vi "PathPlanner_Trajectory25_GenerateStates_Pass1.vi"(8 "StartingRotation":T5={"VALUE"=0.0, "COS"=1.0, "SIN"=0.0} {"SIN" format="%13.4f"; "COS" format="%13.4f"; "VALUE" format="%13.4f"}, 9 "RobotConfig":T1 {"moduleLocations"."Y" format="%14.3f"; "moduleLocations"."X" format="%14.3f"; "ModuleConfig"."driveMotor"."Jr_KgM2" format="%13.5p"; "ModuleConfig"."driveMotor"."L_H" format="%13.5p"; "ModuleConfig"."driveMotor"."Kt_NMPerAmp" format="%13.5p"; "ModuleConfig"."driveMotor"."KvINV_RadPerSecPerVolt" format="%13.5p"; "ModuleConfig"."driveMotor"."R_Ohms" format="%13.5p"; "ModuleConfig"."driveMotor"."FreeSpeed_RadPerSec" format="%13.5p"; "ModuleConfig"."driveMotor"."FreeCurrent_Amps" format="%13.5p"; "ModuleConfig"."driveMotor"."StallCurrent_Amps" format="%13.5p"; "ModuleConfig"."driveMotor"."StallTorque_NM" format="%13.5p"; "ModuleConfig"."driveMotor"."nominalVoltage_Volts" format="%13.5p"}, 10 "in PathPlannerStates":T6[](array[typedef]) {"ModuleStates"."SWERVE_DRIVE_MODULE_STATE"."Angle"."SIN" format="%13.4f"; "ModuleStates"."SWERVE_DRIVE_MODULE_STATE"."Angle"."COS" format="%13.4f"; "ModuleStates"."SWERVE_DRIVE_MODULE_STATE"."Angle"."VALUE" format="%13.4f"; "ModuleStates"."FieldAngle"."SIN" format="%13.4f"; "ModuleStates"."FieldAngle"."COS" format="%13.4f"; "ModuleStates"."FieldAngle"."VALUE" format="%13.4f"; "ModuleStates"."FieldPos"."Y" format="%14.3f"; "ModuleStates"."FieldPos"."X" format="%14.3f"; "DeltaRot"."SIN" format="%13.4f"; "DeltaRot"."COS" format="%13.4f"; "DeltaRot"."VALUE" format="%13.4f"; "pose"."ROTATION"."SIN" format="%13.4f"; "pose"."ROTATION"."COS" format="%13.4f"; "pose"."ROTATION"."VALUE" format="%13.4f"; "pose"."TRANSLATION"."Y" format="%14.3f"; "pose"."TRANSLATION"."X" format="%14.3f"; "FieldSpeeds"."vOmega" format="%10.3f"; "FieldSpeeds"."vY" format="%10.3f"; "FieldSpeeds"."vX" format="%10.3f"; "Heading"."SIN" format="%13.4f"; "Heading"."COS" format="%13.4f"; "Heading"."VALUE" format="%13.4f"}, 11 "PathPlannerPath":T13={"Reversed"=FALSE, "RotationTargets"=[], "ConstraintZones"=[], "EventMarkers"=[], "GlobalConstraints"={"MaxVelocityMps;"=0.0, "MaxAccelerationMpsSq;"=0.0, "MaxAngularVelRadPsEc;"=0.0, "MaxAngularAccRadPSecSq"=0.0, "Exists"=FALSE, "Unlimited"=FALSE, "NominalVoltageVolts"=12.0}, "GoalEndState"={"VelocityMPS"=0.0, "Rotation"={"VALUE"=0.0, "COS"=1.0, "SIN"=0.0}}, "AllPoints"=[], "Name"="", "Waypoints"=[], "PointTowardsZones"=[], "IdealStartingState"={"VelocityMPS"=0.0, "Rotation"={"VALUE"=1.0, "COS"=0.0, "SIN"=0.0}}, "IsChoreoPath"=FALSE, "PreventFlipping"=FALSE} {"IdealStartingState"."Rotation"."SIN" format="%13.4f"; "IdealStartingState"."Rotation"."COS" format="%13.4f"; "IdealStartingState"."Rotation"."VALUE" format="%13.4f"; "PointTowardsZones"."TargetPosition"."Y" format="%14.3f"; "PointTowardsZones"."TargetPosition"."X" format="%14.3f"; "PointTowardsZones"."RotationOffset"."SIN" format="%13.4f"; "PointTowardsZones"."RotationOffset"."COS" format="%13.4f"; "PointTowardsZones"."RotationOffset"."VALUE" format="%13.4f"; "Waypoints"."nextControl"."Y" format="%14.3f"; "Waypoints"."nextControl"."X" format="%14.3f"; "Waypoints"."anchor"."Y" format="%14.3f"; "Waypoints"."anchor"."X" format="%14.3f"; "Waypoints"."prevControl"."Y" format="%14.3f"; "Waypoints"."prevControl"."X" format="%14.3f"; "AllPoints"."RotationTarget"."rotation"."SIN" format="%13.4f"; "AllPoints"."RotationTarget"."rotation"."COS" format="%13.4f"; "AllPoints"."RotationTarget"."rotation"."VALUE" format="%13.4f"; "AllPoints"."Position"."Y" format="%14.3f"; "AllPoints"."Position"."X" format="%14.3f"; "GoalEndState"."Rotation"."SIN" format="%13.4f"; "GoalEndState"."Rotation"."COS" format="%13.4f"; "GoalEndState"."Rotation"."VALUE" format="%13.4f"; "RotationTargets"."rotation"."SIN" format="%13.4f"; "RotationTargets"."rotation"."COS" format="%13.4f"; "RotationTargets"."rotation"."VALUE" format="%13.4f"}) -> (3 "out PathPlannerStates":T6[](array[typedef]) {"ModuleStates"."SWERVE_DRIVE_MODULE_STATE"."Angle"."SIN" format="%13.4f"; "ModuleStates"."SWERVE_DRIVE_MODULE_STATE"."Angle"."COS" format="%13.4f"; "ModuleStates"."SWERVE_DRIVE_MODULE_STATE"."Angle"."VALUE" format="%13.4f"; "ModuleStates"."FieldAngle"."SIN" format="%13.4f"; "ModuleStates"."FieldAngle"."COS" format="%13.4f"; "ModuleStates"."FieldAngle"."VALUE" format="%13.4f"; "ModuleStates"."FieldPos"."Y" format="%14.3f"; "ModuleStates"."FieldPos"."X" format="%14.3f"; "DeltaRot"."SIN" format="%13.4f"; "DeltaRot"."COS" format="%13.4f"; "DeltaRot"."VALUE" format="%13.4f"; "pose"."ROTATION"."SIN" format="%13.4f"; "pose"."ROTATION"."COS" format="%13.4f"; "pose"."ROTATION"."VALUE" format="%13.4f"; "pose"."TRANSLATION"."Y" format="%14.3f"; "pose"."TRANSLATION"."X" format="%14.3f"; "FieldSpeeds"."vOmega" format="%10.3f"; "FieldSpeeds"."vY" format="%10.3f"; "FieldSpeeds"."vX" format="%10.3f"; "Heading"."SIN" format="%13.4f"; "Heading"."COS" format="%13.4f"; "Heading"."VALUE" format="%13.4f"})   [LabVIEW 2019, in "PathPlanner24.lvlib"]
doc: "Internal routine to help create a trajectory from a path."
uses:
  PathPlanner24.lvlib
  TypeDef/PathPlannerTrajectoryState25.ctl
  <vilib>/Rock Robotics/WPI/ThirdParty/JAS_Junk/TrajLib/TypeDef/ROTATION2D.ctl
  TypeDef/PathPlannerPathConstraints.ctl
  <vilib>/Rock Robotics/WPI/ThirdParty/JAS_Junk/TrajLib/TypeDef/CHASSIS_SPEEDS.ctl
  <vilib>/Rock Robotics/WPI/ThirdParty/JAS_Junk/TrajLib/TypeDef/POSE2D.ctl
  <vilib>/Rock Robotics/WPI/ThirdParty/JAS_Junk/TrajLib/TypeDef/TRANSLATION2D.ctl
  TypeDef/PathPlannerSwerveModTrajState.ctl
  <vilib>/Rock Robotics/WPI/ThirdParty/JAS_Junk/TrajLib/TypeDef/SWERVE_DRIVE_MODULE_STATE.ctl
  TypeDef/PathPlannerDriveFeedFwds.ctl
  TypeDef/PathPlannerPath.ctl
  TypeDef/PathPlannerRotationTarget.ctl
  TypeDef/PathPlannerConstraintsZone.ctl
  TypeDef/PathPlannerEventMarker.ctl
  TypeDef/PathPlannerCommandUtil.ctl
  ENum/PathPlanner_CommandUtilType_ENUM.ctl
  TypeDef/PathPlannerGoalEndState.ctl
  TypeDef/PathPlannerPathPoint.ctl
  TypeDef/PathPlannerWaypoint.ctl
  TypeDef/PathPlannerPointTowardsZone.ctl
  TypeDef/PathPlannerIdealStartingState.ctl
  TypeDef/PathPlannerRobotConfig.ctl
  TypeDef/PathPlannerModuleConfig.ctl
  <vilib>/Rock Robotics/WPI/ThirdParty/JAS_Junk/TrajLib/TypeDef/DCMOTOR.CTL
  PathPlanner_GeomUtil_RotationLerp.vi
  <vilib>/Rock Robotics/WPI/ThirdParty/JAS_Junk/TrajLib/Translation2d_Create.vi
  <vilib>/Rock Robotics/WPI/ThirdParty/JAS_Junk/TrajLib/Util_CalcDist.vi
  <vilib>/Rock Robotics/WPI/ThirdParty/JAS_Junk/TrajLib/Translation2d_GetXY.vi
  <vilib>/Rock Robotics/WPI/ThirdParty/JAS_Junk/TrajLib/Rotation2d_CreateXY.vi
  <vilib>/Rock Robotics/WPI/ThirdParty/JAS_Junk/TrajLib/Conv_Deg_Radians.vi
  <vilib>/Rock Robotics/WPI/ThirdParty/JAS_Junk/TrajLib/Rotation2d_RotateBy.vi
  <vilib>/Rock Robotics/WPI/ThirdParty/JAS_Junk/TrajLib/Rotation2d_UnaryMinus.vi
  <vilib>/Rock Robotics/WPI/ThirdParty/JAS_Junk/TrajLib/Rotation2d_Times.vi
  <vilib>/Rock Robotics/WPI/ThirdParty/JAS_Junk/TrajLib/Trajectory_Library.lvlib
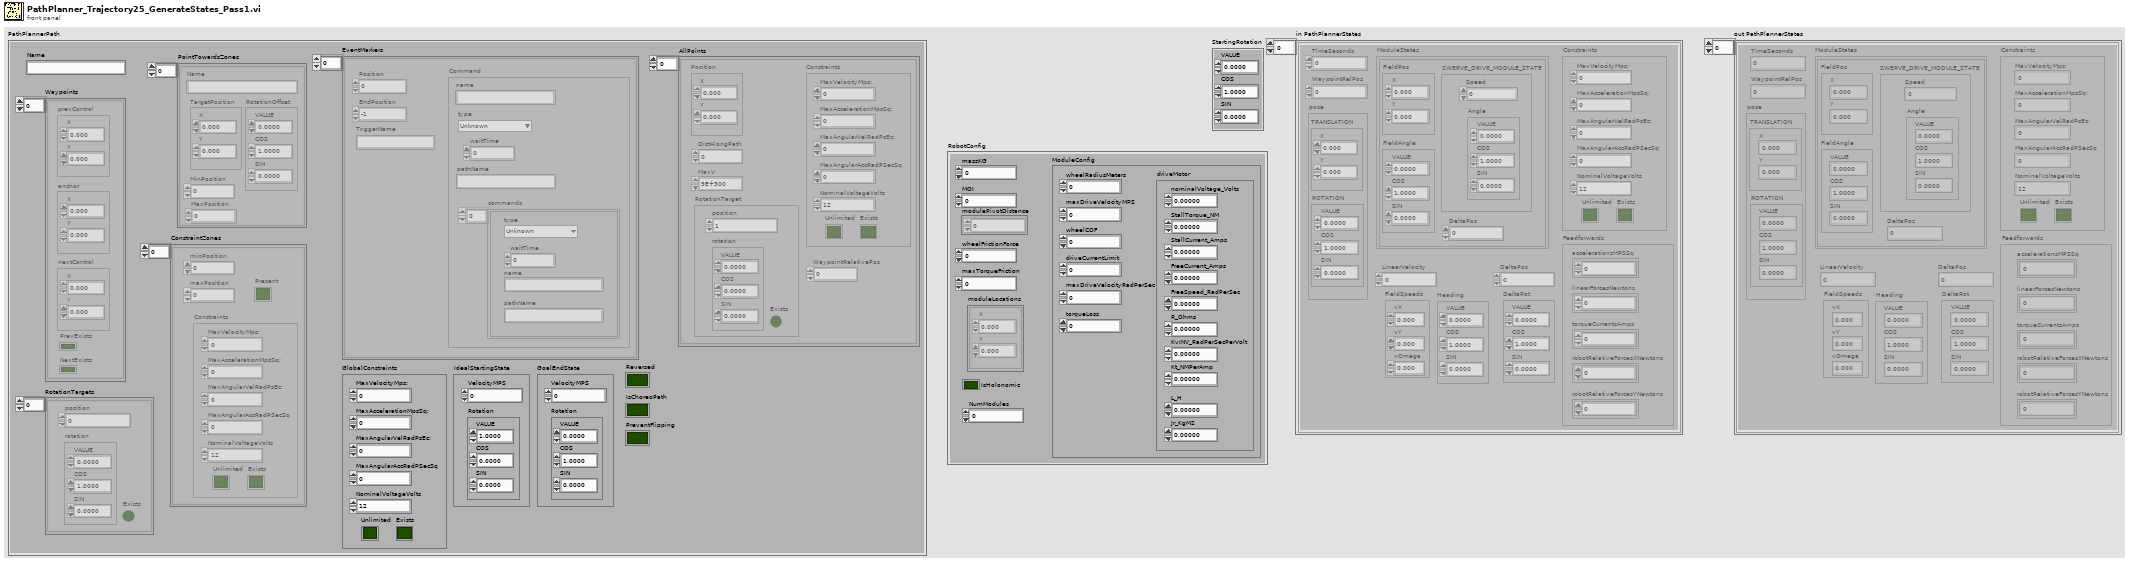
[diagram p1: front panel]
types:
  T1 = typedef "PathPlanner24.lvlib/PathPlannerRobotConfig.ctl" = cluster{"massKG":dbl, "MOI":dbl, "modulePivotDistance":dbl[], "wheelFrictionForce":dbl, "maxTorqueFriction":dbl, "ModuleConfig":T2, "moduleLocations":T4[], "IsHolonomic":bool, "NumModules":i32}
  T2 = typedef "PathPlanner24.lvlib/PathPlannerModuleConfig.ctl" = cluster{"wheelRadiusMeters":dbl, "maxDriveVelocityMPS":dbl, "wheelCOF":dbl, "driveCurrentLimit":dbl, "maxDriveVelocityRadPerSec":dbl, "torqueLoss":dbl, "driveMotor":T3}
  T3 = typedef "Trajectory_Library.lvlib/DCMOTOR.CTL" = cluster{"nominalVoltage_Volts":dbl, "StallTorque_NM":dbl, "StallCurrent_Amps":dbl, "FreeCurrent_Amps":dbl, "FreeSpeed_RadPerSec":dbl, "R_Ohms":dbl, "KvINV_RadPerSecPerVolt":dbl, "Kt_NMPerAmp":dbl, "L_H":dbl, "Jr_KgM2":dbl}
  T4 = typedef "Trajectory_Library.lvlib/TRANSLATION2D.ctl" = cluster{"X":dbl, "Y":dbl}
  T5 = typedef "Trajectory_Library.lvlib/ROTATION2D.ctl" = cluster{"VALUE":dbl, "COS":dbl, "SIN":dbl}
  T6 = typedef "PathPlanner24.lvlib/PathPlannerTrajectoryState25.ctl" = cluster{"TimeSeconds":dbl, "LinearVelocity":dbl, "Heading":T5, "Constraints":T7, "DeltaPos":dbl, "FieldSpeeds":T8, "pose":T9, "DeltaRot":T5, "ModuleStates":T10[], "WaypointRelPos":dbl, "Feedforwards":T12}
  T7 = typedef "PathPlanner24.lvlib/PathPlannerPathConstraints.ctl" = cluster{"MaxVelocityMps;":dbl, "MaxAccelerationMpsSq;":dbl, "MaxAngularVelRadPsEc;":dbl, "MaxAngularAccRadPSecSq":dbl, "Exists":bool, "Unlimited":bool, "NominalVoltageVolts":dbl}
  T8 = typedef "Trajectory_Library.lvlib/CHASSIS_SPEEDS.ctl" = cluster{"vX":dbl, "vY":dbl, "vOmega":dbl}
  T9 = typedef "Trajectory_Library.lvlib/POSE2D.ctl" = cluster{"TRANSLATION":T4, "ROTATION":T5}
  T10 = typedef "PathPlanner24.lvlib/PathPlannerSwerveModTrajState.ctl" = cluster{"FieldPos":T4, "FieldAngle":T5, "DeltaPos":dbl, "SWERVE_DRIVE_MODULE_STATE":T11}
  T11 = typedef "Trajectory_Library.lvlib/SWERVE_DRIVE_MODULE_STATE.ctl" = cluster{"Speed":dbl, "Angle":T5}
  T12 = typedef "PathPlanner24.lvlib/PathPlannerDriveFeedFwds.ctl" = cluster{"accelerationsMPSSq":dbl[], "linearForcesNewtons":dbl[], "torqueCurrentsAmps":dbl[], "robotRelativeForcesXNewtons":dbl[], "robotRelativeForcesYNewtons":dbl[]}
  T13 = typedef "PathPlanner24.lvlib/PathPlannerPath.ctl" = cluster{"Reversed":bool, "RotationTargets":T14[], "ConstraintZones":T15[], "EventMarkers":T16[], "GlobalConstraints":T7, "GoalEndState":T19, "AllPoints":T20[], "Name":string, "Waypoints":T21[], "PointTowardsZones":T22[], "IdealStartingState":T23, "IsChoreoPath":bool, "PreventFlipping":bool}
  T14 = typedef "PathPlanner24.lvlib/PathPlannerRotationTarget.ctl" = cluster{"position":dbl, "rotation":T5, "Exists":bool}
  T15 = typedef "PathPlanner24.lvlib/PathPlannerConstraintsZone.ctl" = cluster{"minPosition":dbl, "maxPosition":dbl, "Constraints":T7, "Present":bool}
  T16 = typedef "PathPlanner24.lvlib/PathPlannerEventMarker.ctl" = cluster{"Position":dbl, "Command":T17, "TriggerName":string, "EndPosition":dbl}
  T17 = typedef "PathPlanner24.lvlib/PathPlannerCommandUtil.ctl" = cluster{"waitTime":dbl, "name":string, "pathName":string, "commands":cluster{"type":T18, "waitTime":dbl, "name":string, "pathName":string}[], "type":T18}
  T18 = typedef "PathPlanner24.lvlib/PathPlanner_CommandUtilType_ENUM.ctl" = enum16{"Unknown", "Wait", "Named", "Path", "Sequential", "Parallel", "Race", "Deadline"}
  T19 = typedef "PathPlanner24.lvlib/PathPlannerGoalEndState.ctl" = cluster{"VelocityMPS":dbl, "Rotation":T5}
  T20 = typedef "PathPlanner24.lvlib/PathPlannerPathPoint.ctl" = cluster{"Position":T4, "DistAlongPath":dbl, "MaxV":dbl, "Constraints":T7, "RotationTarget":T14, "WaypointRelativePos":dbl}
  T21 = typedef "PathPlanner24.lvlib/PathPlannerWaypoint.ctl" = cluster{"prevControl":T4, "anchor":T4, "nextControl":T4, "PrevExists":bool, "NextExists":bool}
  T22 = typedef "PathPlanner24.lvlib/PathPlannerPointTowardsZone.ctl" = cluster{"RotationOffset":T5, "Name":string, "TargetPosition":T4, "MinPosition":dbl, "MaxPosition":dbl}
  T23 = typedef "PathPlanner24.lvlib/PathPlannerIdealStartingState.ctl" = cluster{"VelocityMPS":dbl, "Rotation":T5}
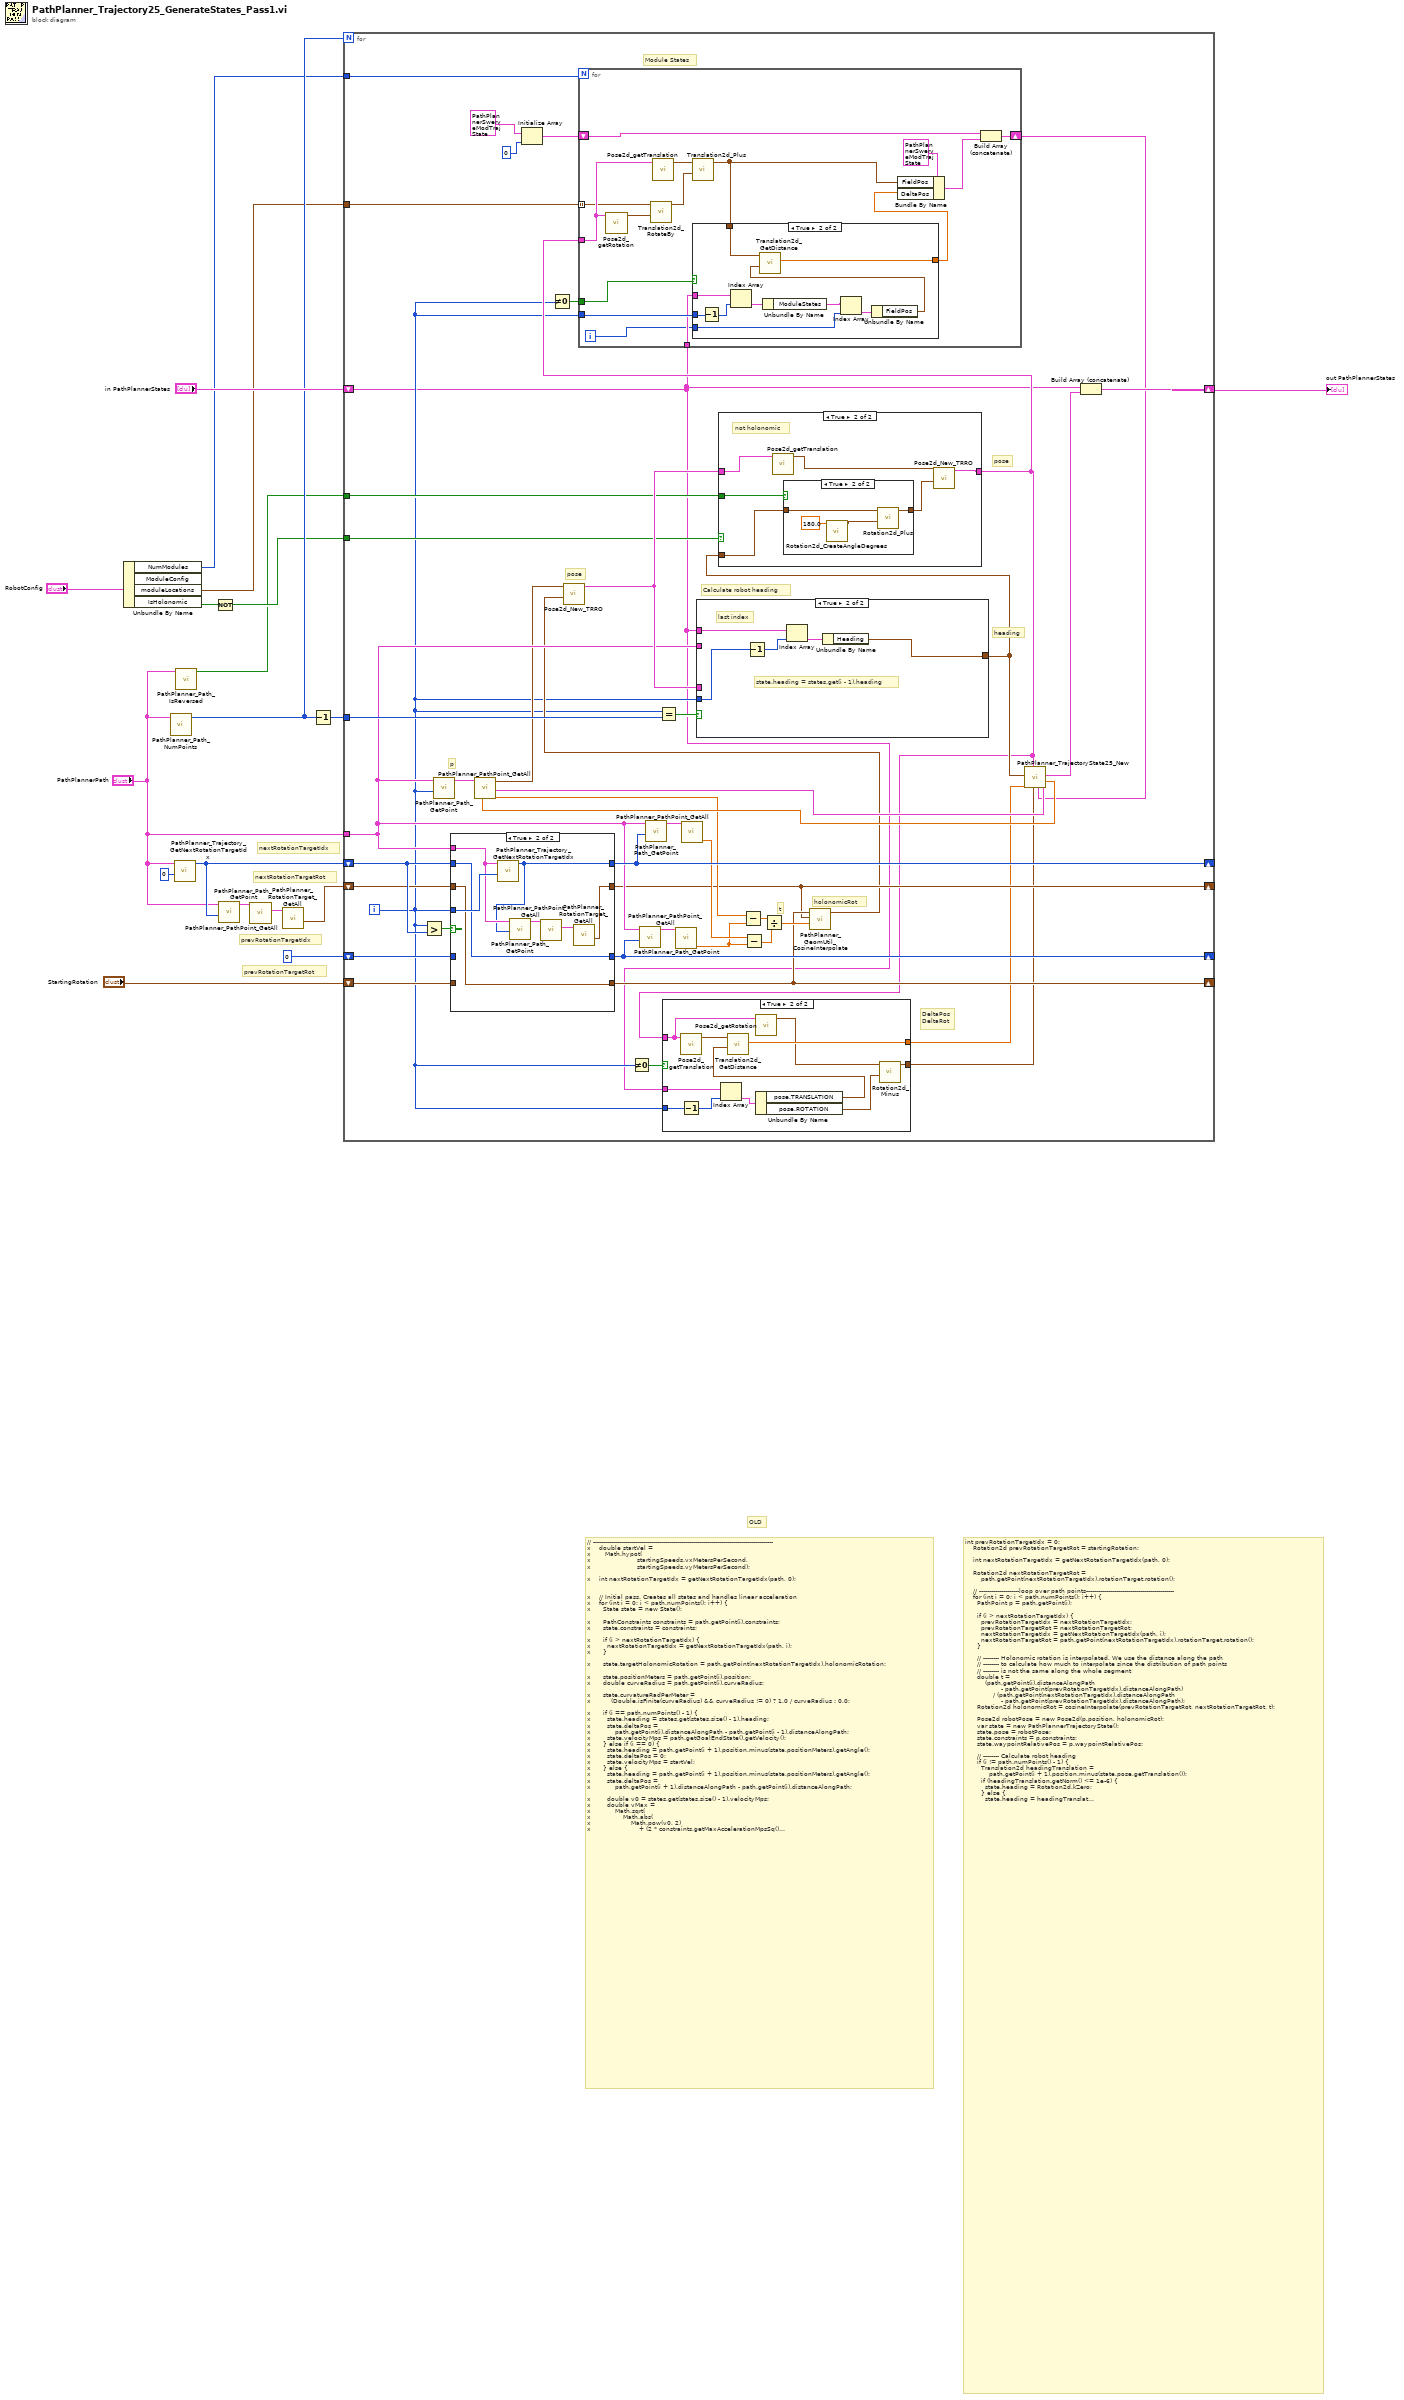
[diagram p0: block diagram]
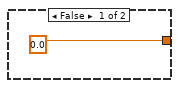
[diagram p2: hidden frame]
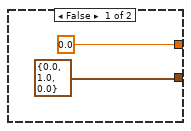
[diagram p3: hidden frame]
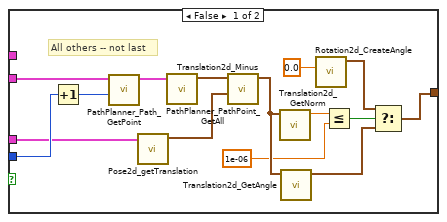
[diagram p6: hidden frame]
diagram:
  # "nextRotationTargetRot"
  # "prevRotationTargetRot"
  # "prevRotationTargetIdx"
  # "nextRotationTargetIdx"
  # "OLD"
  # "int prevRotationTargetIdx = 0;\n    Rotation2d prevRotationTargetRot = startingRotation;\n\n    int nextRotationTargetIdx = getNextRotationTargetIdx(path, 0);\n\n    Rotation2d nextRotationTargetRot =\n        path.getPoint(nextRotationTargetIdx).rotationTarget.rotation();\n\n    // --------------------loop over path points--------------------------------------------\n    for (int i = 0; i < path.numPoints(); i++) {\n      PathPoint p = path.getPoint(i);\n\n      if (i > nextRotationTargetIdx) {\n        prevRotationTargetIdx = nextRotationTargetIdx;\n        prevRotationTargetRot = nextRotationTargetRot;\n        nextRotationTargetIdx = getNextRotationTargetIdx(path, i);\n        nextRotationTargetRot = path.getPoint(nextRotationTargetIdx).rotationTarget.rotation();\n      }\n\n      // -------- Holonomic rotation is interpolated. We use the distance along the path\n      // -------- to calculate how much to interpolate since the distribution of path points\n      // -------- is not the same along the whole segment\n      double t =\n          (path.getPoint(i).distanceAlongPath\n                  - path.getPoint(prevRotationTargetIdx).distanceAlongPath)\n              / (path.getPoint(nextRotationTargetIdx).distanceAlongPath\n                  - path.getPoint(prevRotationTargetIdx).distanceAlongPath);\n      Rotation2d holonomicRot = cosineInterpolate(prevRotationTargetRot, nextRotationTargetRot, t);\n\n      Pose2d robotPose = new Pose2d(p.position, holonomicRot);\n      var state = new PathPlannerTrajectoryState();\n      state.pose = robotPose;\n      state.constraints = p.constraints;\n      state.waypointRelativePos = p.waypointRelativePos;\n\n      // -------- Calculate robot heading\n      if (i != path.numPoints() - 1) {\n        Translation2d headingTranslation =\n            path.getPoint(i + 1).position.minus(state.pose.getTranslation());\n        if (headingTranslation.getNorm() <= 1e-6) {\n          state.heading = Rotation2d.kZero;\n        } else {\n          state.heading = headingTranslation.getAngle();\n        }\n      } else {\n        state.heading = states.get(i - 1).heading;\n      }\n\n      if (!config.isHolonomic) {\n        state.pose =\n            new Pose2d(\n                state.pose.getTranslation(),\n                path.isReversed() ? (state.heading.plus(Rotation2d.k180deg)) : state.heading);\n      }\n\n      if (i != 0) {\n        state.deltaPos =\n            state.pose.getTranslation().getDistance(states.get(i - 1).pose.getTranslation());\n        state.deltaRot = state.pose.getRotation().minus(states.get(i - 1).pose.getRotation());\n      }\n\n      state.moduleStates = new SwerveModuleTrajectoryState[config.numModules];\n      // -------------------------inner loop---------------------------------------\n      for (int m = 0; m < config.numModules; m++) {\n        state.moduleStates[m] = new SwerveModuleTrajectoryState();\n        state.moduleStates[m].fieldPos =\n            state\n                .pose\n                .getTranslation()\n                .plus(config.moduleLocations[m].rotateBy(state.pose.getRotation()));\n\n        if (i != 0) {\n          state.moduleStates[m].deltaPos =\n              state.moduleStates[m].fieldPos.getDistance(\n                  states.get(i - 1).moduleStates[m].fieldPos);\n        }\n      }\n      // ----------------------------end inner loop---------------------------------\n      states.add(state);\n    }\n    // -------------------------------end loop-----------------------------------------------------"
  # "// ------------------------------------------------------------------------------------------\nx    double startVel =\nx       Math.hypot(  \nx                       startingSpeeds.vxMetersPerSecond, \nx                       startingSpeeds.vyMetersPerSecond);\n\nx    int nextRotationTargetIdx = getNextRotationTargetIdx(path, 0);\n\n\nx    // Initial pass. Creates all states and handles linear acceleration\nx    for (int i = 0; i < path.numPoints(); i++) {\nx      State state = new State();\n\nx      PathConstraints constraints = path.getPoint(i).constraints;\nx      state.constraints = constraints;\n\nx      if (i > nextRotationTargetIdx) {\nx        nextRotationTargetIdx = getNextRotationTargetIdx(path, i);\nx      }\n\nx      state.targetHolonomicRotation = path.getPoint(nextRotationTargetIdx).holonomicRotation;\n\nx      state.positionMeters = path.getPoint(i).position;\nx      double curveRadius = path.getPoint(i).curveRadius;\n\nx      state.curvatureRadPerMeter =\nx          (Double.isFinite(curveRadius) && curveRadius != 0) ? 1.0 / curveRadius : 0.0;\n\nx      if (i == path.numPoints() - 1) {\nx        state.heading = states.get(states.size() - 1).heading;\nx        state.deltaPos =\nx            path.getPoint(i).distanceAlongPath - path.getPoint(i - 1).distanceAlongPath;\nx        state.velocityMps = path.getGoalEndState().getVelocity();\nx      } else if (i == 0) {\nx        state.heading = path.getPoint(i + 1).position.minus(state.positionMeters).getAngle();\nx        state.deltaPos = 0;\nx        state.velocityMps = startVel;\nx      } else {\nx        state.heading = path.getPoint(i + 1).position.minus(state.positionMeters).getAngle();\nx        state.deltaPos =\nx            path.getPoint(i + 1).distanceAlongPath - path.getPoint(i).distanceAlongPath;\n\nx        double v0 = states.get(states.size() - 1).velocityMps;\nx        double vMax =\nx            Math.sqrt(\nx                Math.abs(\nx                    Math.pow(v0, 2)\nx                        + (2 * constraints.getMaxAccelerationMpsSq() * state.deltaPos)));\nx        state.velocityMps = Math.min(vMax, path.getPoint(i).maxV);\n      }\n\nX      states.add(state);\n    }"
  n1 = Unbundle By Name("RobotConfig") -> ("NumModules"=w2:i32, "moduleLocations"=w1:T4[], "IsHolonomic"=w6:bool)  [unwired: 1 out]
  n2 = call "PathPlanner_Path_NumPoints.vi"("PathPlannerPath"="PathPlannerPath") -> ("NumPoints"=w14:i32)  [unwired: 10 in]
  n3 = call "PathPlanner_Trajectory_GetNextRotationTargetIdx.vi"("Starting Index"=0, "PathPlannerPath"="PathPlannerPath") -> ("Idx"=w8:i32)  [unwired: 8 in, 1 out]
  n4 = call "PathPlanner_Path_IsReversed.vi"("PathPlannerPath"="PathPlannerPath") -> ("Reversed"=w3:bool)  [unwired: 10 in]
  n5 = Not(x=w6) -> (.not. x?=w5:bool)
  n6 = call "PathPlanner_Path_GetPoint.vi"("Index"=w8, "PathPlannerPath"="PathPlannerPath") -> ("Point"=w9:T20)  [unwired: 9 in]
  n7 = call "PathPlanner_PathPoint_GetAll.vi"("PathPlannerPoint"=w9) -> ("RotationTarget"=w11:T14)  [unwired: 5 in, 5 out]
  n8 = call "PathPlanner_RotationTarget_GetAll.vi"("RotationTarget"=w11) -> ("rotation"=w10:T5)  [unwired: 8 in, 2 out]
  n9 = Decrement(x=w14) -> (x-1=w15:i32)
  n10 = for {
    N: w14 -> [_]
    shift-right: [w62] -> w17
    shift-left: "in PathPlannerStates" -> [w19]
    shift-right: [w59] -> _
    shift-left: w8 -> [w60]
    tunnel: "PathPlannerPath" -> [w46]
    tunnel: w15 -> [w57]
    shift-right: [w45] -> _
    shift-left: 0 ("Starting Index") -> [w52]
    shift-right: [w37] -> _
    shift-left: "StartingRotation" -> [w51]
    shift-right: [w36] -> _
    shift-left: w10 -> [w50]
    tunnel: w5 -> [w33]
    tunnel: w3 -> [w32]
    tunnel: w2 -> [w28]
    tunnel: w1 -> [w23]
    i -> [w20]
    # "Module States"
    # "DeltaPos\nDeltaRot"
    # "holonomicRot"
    # "t"
    # "heading"
    # "pose"
    # "pose"
    # "Calculate robot heading"
    # "p"
    n11 = Greater?(x=w20, y=w60) -> (0:w61:bool)
    n12 = call "PathPlanner_Path_GetPoint.vi"("Index"=w20, "PathPlannerPath"=w46) -> ("Point"=w53:T20)  [unwired: 9 in]
    n13 = case shown="True" w61 {
      tunnel: w20 -> [_ w145]
      tunnel: w46 -> [_ w142]
      tunnel: [w137 w141] -> w59
      tunnel: w60 -> [w137 w139]
      tunnel: w52 -> [w136 _]
      tunnel: w51 -> [w135 _]
      tunnel: [w136 w139] -> w45
      tunnel: [w135 w138] -> w37
      tunnel: w50 -> [w134 w138]
      tunnel: [w134 w140] -> w36
      frame False {
      }
      frame True {
        n14 = call "PathPlanner_Trajectory_GetNextRotationTargetIdx.vi"("Starting Index"=w145, "PathPlannerPath"=w142) -> ("Idx"=w141:i32)  [unwired: 8 in, 1 out]
        n15 = call "PathPlanner_Path_GetPoint.vi"("Index"=w141, "PathPlannerPath"=w142) -> ("Point"=w143:T20)  [unwired: 9 in]
        n16 = call "PathPlanner_PathPoint_GetAll.vi"("PathPlannerPoint"=w143) -> ("RotationTarget"=w144:T14)  [unwired: 5 in, 5 out]
        n17 = call "PathPlanner_RotationTarget_GetAll.vi"("RotationTarget"=w144) -> ("rotation"=w140:T5)  [unwired: 8 in, 2 out]
      }
    }
    n18 = call "PathPlanner_PathPoint_GetAll.vi"("PathPlannerPoint"=w53) -> ("DistAlongPath"=w42:dbl, "Constraints"=w54:T7, "Position"=w34:T4, "WaypointRelativePos"=w49:dbl)  [unwired: 5 in, 2 out]
    n19 = Initialize Array(T10 {"FieldPos"={"X"=0.0, "Y"=0.0}, "FieldAngle"={"VALUE"=0.0, "COS"=1.0, "SIN"=0.0}, "DeltaPos"=0.0, "SWERVE_DRIVE_MODULE_STATE"={"Speed"=0.0, "Angle"={"VALUE"=0.0, "COS"=1.0, "SIN"=0.0}}} ("PathPlannerSwerveModuleTrajectoryState"), 0 ("dimension size")) -> (w25:T10[])
    n20 = Not Equal To 0?(x=w20) -> (x != 0?=w21:bool)
    n21 = Not Equal To 0?(x=w20) -> (x != 0?=w31:bool)
    n22 = call "PathPlanner_Path_GetPoint.vi"("Index"=w45, "PathPlannerPath"=w46) -> ("Point"=w44:T20)  [unwired: 9 in]
    n23 = call "PathPlanner_Path_GetPoint.vi"("Index"=w59, "PathPlannerPath"=w46) -> ("Point"=w58:T20)  [unwired: 9 in]
    n24 = Equal?(x=w20, y=w57) -> (x = y?=w56:bool)
    n25 = call "PathPlanner_PathPoint_GetAll.vi"("PathPlannerPoint"=w44) -> ("DistAlongPath"=w40:dbl)  [unwired: 5 in, 5 out]
    n26 = call "PathPlanner_PathPoint_GetAll.vi"("PathPlannerPoint"=w58) -> ("DistAlongPath"=w41:dbl)  [unwired: 5 in, 5 out]
    n27 = Subtract(x=w42, y=w40) -> (x-y=w43:dbl)
    n28 = Subtract(x=w41, y=w40) -> (x-y=w39:dbl)
    n29 = Divide(x=w43, y=w39) -> (x/y=w38:dbl)
    n30 = call "PathPlanner_GeomUtil_CosineInterpolate.vi"("T"=w38, "EndVal"=w36, "StartVal"=w37) -> ("InterpolatedValue"=w35:T5)  [unwired: 8 in]
    n31 = call <vilib>:"Pose2d_New_TRRO.vi"("ROTATION"=w35, "TRANSLATION"=w34) -> ("outPOSE"=w48:T9)  [unwired: 9 in]
    n32 = case shown="True" w56 {
      tunnel: w20 -> [w128 w131]
      tunnel: w19 -> [_ w133]
      tunnel: [w116 w129] -> w47
      tunnel: w46 -> [w124 _]
      tunnel: w48 -> [w115 _]
      frame False {
        # "All others -- not last"
        n33 = Increment(x=w128) -> (x+1=w126:i32)
        n34 = call "PathPlanner_Path_GetPoint.vi"("Index"=w126, "PathPlannerPath"=w124) -> ("Point"=w127:T20)  [unwired: 9 in]
        n35 = call <vilib>:"Pose2d_getTranslation.vi"("in POSE"=w115) -> ("outTRANSLATION"=w114:T4)  [unwired: 10 in]
        n36 = call "PathPlanner_PathPoint_GetAll.vi"("PathPlannerPoint"=w127) -> ("Position"=w125:T4)  [unwired: 5 in, 5 out]
        n37 = call <vilib>:"Translation2d_Minus.vi"("other Translation"=w114, "In Translation"=w125) -> ("Out Translation"=w123:T4)  [unwired: 9 in]
        n38 = call <vilib>:"Translation2d_GetNorm.vi"("In Translation"=w123) -> ("Norm"=w122:dbl)  [unwired: 10 in]
        n39 = call <vilib>:"Translation2d_GetAngle.vi"("In Translation"=w123) -> ("Angle_Rotation2d"=w119:T5)  [unwired: 10 in]
        n40 = call <vilib>:"Rotation2d_CreateAngle.vi"("Angle"=0.0) -> ("ROTATION"=w117:T5)  [unwired: 10 in]
        n41 = Less Or Equal?(x=w122, y=1e-06) -> (x <= y?=w120:bool)
        n42 = Select(t=w117, s=w120, f=w119) -> (s? t:f=w116:T5)
      }
      frame True {
        # "state.heading = states.get(i - 1).heading"
        # "last index"
        n43 = Decrement(x=w131) -> (x-1=w132:i32)
        n44 = Index Array(array=w133, index=w132) -> (element=w130:T6)
        n45 = Unbundle By Name(w130) -> ("Heading"=w129:T5)
      }
    }
    n46 = case shown="True" w33 {
      tunnel: w48 -> [w102 w108]
      tunnel: [w102 w104] -> w24
      tunnel: w47 -> [_ w106]
      tunnel: w32 -> [_ w103]
      frame False {
      }
      frame True {
        # "not holonomic"
        n47 = call <vilib>:"Pose2d_getTranslation.vi"("in POSE"=w108) -> ("outTRANSLATION"=w107:T4)  [unwired: 10 in]
        n48 = case shown="True" w103 {
          tunnel: w106 -> [w109 w112]
          tunnel: [w109 w113] -> w105
          frame False {
          }
          frame True {
            n49 = call <vilib>:"Rotation2d_CreateAngleDegrees.vi"("Angle_Degrees"=180.0) -> ("ROTATION"=w110:T5)  [unwired: 10 in]
            n50 = call <vilib>:"Rotation2d_Plus.vi"("other ROTATION"=w110, "in ROTATION"=w112) -> ("out ROTATION"=w113:T5)  [unwired: 9 in]
          }
        }
        n51 = call <vilib>:"Pose2d_New_TRRO.vi"("ROTATION"=w105, "TRANSLATION"=w107) -> ("outPOSE"=w104:T9)  [unwired: 9 in]
      }
    }
    n52 = for {
      N: w28 -> [_]
      shift-right: [w74] -> w22
      shift-left: w25 -> [w75]
      tunnel: w24 -> [w73]
      tunnel: w23 -> [w70] mode=indexing
      tunnel: w21 -> [w68]
      tunnel: w20 -> [w66]
      tunnel: w19 -> [w65]
      i -> [w64]
      n53 = call <vilib>:"Pose2d_getRotation.vi"("in POSE"=w73) -> ("out ROTATION"=w72:T5)  [unwired: 10 in]
      n54 = call <vilib>:"Translation2d_RotateBy.vi"("other Rotation"=w72, "In Translation"=w70) -> ("Out Translation"=w69:T4)  [unwired: 9 in]
      n55 = call <vilib>:"Pose2d_getTranslation.vi"("in POSE"=w73) -> ("outTRANSLATION"=w71:T4)  [unwired: 10 in]
      n56 = call <vilib>:"Translation2d_Plus.vi"("other Translation"=w69, "In Translation"=w71) -> ("Out Translation"=w67:T4)  [unwired: 9 in]
      n57 = case shown="True" w68 {
        tunnel: w67 -> [_ w88]
        tunnel: w66 -> [_ w86]
        tunnel: w65 -> [_ w85]
        tunnel: w64 -> [_ w82]
        tunnel: [0.0 w79] -> w63
        frame False {
        }
        frame True {
          n58 = Decrement(x=w86) -> (x-1=w87:i32)
          n59 = Index Array(array=w85, index=w87) -> (element=w84:T6)
          n60 = Unbundle By Name(w84) -> ("ModuleStates"=w83:T10[])
          n61 = Index Array(array=w83, index=w82) -> (element=w81:T10)
          n62 = Unbundle By Name(w81) -> ("FieldPos"=w80:T4)
          n63 = call <vilib>:"Translation2d_GetDistance.vi"("other Translation"=w80, "In Translation"=w88) -> ("Distance"=w79:dbl)  [unwired: 9 in]
        }
      }
      n64 = Bundle By Name(cluster=T10 {"FieldPos"={"X"=0.0, "Y"=0.0}, "FieldAngle"={"VALUE"=0.0, "COS"=1.0, "SIN"=0.0}, "DeltaPos"=0.0, "SWERVE_DRIVE_MODULE_STATE"={"Speed"=0.0, "Angle"={"VALUE"=0.0, "COS"=1.0, "SIN"=0.0}}} ("PathPlannerSwerveModuleTrajectoryState"), "FieldPos"=w67, "DeltaPos"=w63) -> (w76:T10)
      n65 = Build Array (concatenate)(w75, w76) -> (w74:T10[])
    }
    n66 = case shown="True" w31 {
      tunnel: w24 -> [_ w95]
      tunnel: w19 -> [_ w99]
      tunnel: [0.0 ("Distance") w96] -> w30
      tunnel: [T5 {"VALUE"=0.0, "COS"=1.0, "SIN"=0.0} ("out ROTATION") w92] -> w29
      tunnel: w20 -> [_ w91]
      frame False {
      }
      frame True {
        n67 = call <vilib>:"Pose2d_getTranslation.vi"("in POSE"=w95) -> ("outTRANSLATION"=w98:T4)  [unwired: 10 in]
        n68 = Decrement(x=w91) -> (x-1=w101:i32)
        n69 = Index Array(array=w99, index=w101) -> (element=w100:T6)
        n70 = call <vilib>:"Pose2d_getRotation.vi"("in POSE"=w95) -> ("out ROTATION"=w94:T5)  [unwired: 10 in]
        n71 = Unbundle By Name(w100) -> ("pose.TRANSLATION"=w97:T4, "pose.ROTATION"=w93:T5)
        n72 = call <vilib>:"Translation2d_GetDistance.vi"("other Translation"=w97, "In Translation"=w98) -> ("Distance"=w96:dbl)  [unwired: 9 in]
        n73 = call <vilib>:"Rotation2d_Minus.vi"("other ROTATION"=w93, "in ROTATION"=w94) -> ("out ROTATION"=w92:T5)  [unwired: 9 in]
      }
    }
    n74 = call "PathPlanner_TrajectoryState25_New.vi"("PathPlannerConstraints"=w54, "WaypointRelPos"=w49, "ModuleStates"=w22, "DeltaRot"=w29, "pose"=w24, "DeltaPos"=w30, "Heading"=w47) -> ("PathPlannerState"=w55:T6)  [unwired: 4 in]
    n75 = Build Array (concatenate)(w19, w55) -> (w62:T6[])
  }
  "out PathPlannerStates" <- w17
